vi "InstrPtr Demo.vi"() -> ()   [LabVIEW 2009]
uses:
  Dummy/Dummy.lvclass
  InstrPtr.lvclass
panel:
  out "*dummy":T1
  # "See block diagram."
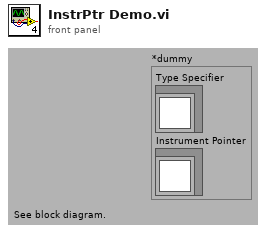
[diagram p1: front panel]
types:
  T1 = cluster{"Type Specifier":refnum<class "Dummy.lvclass">, "Instrument Pointer":refnum<class "InstrPtr.lvclass">}
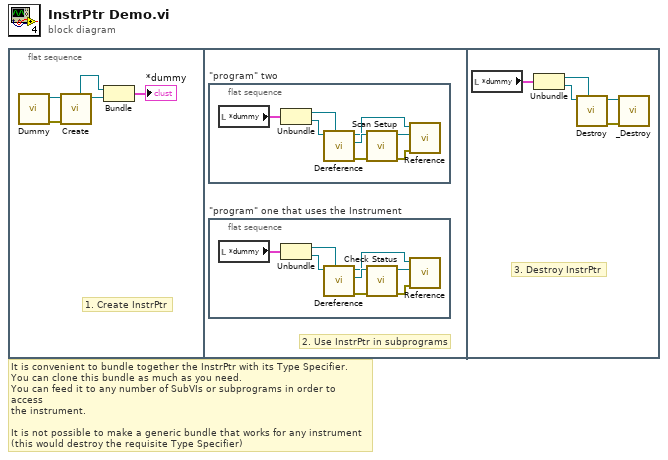
[diagram p0: block diagram]
diagram:
  # "It is convenient to bundle together the InstrPtr with its Type Specifier.\nYou can clone this bundle as much as you need.\nYou can feed it to any number of SubVIs or subprograms in order to access\nthe instrument.\n\nIt is not possible to make a generic bundle that works for any instrument\n(this would destroy the requisite Type Specifier)"
  n1 = flat-sequence {
    frame #0 {
      # "1. Create InstrPtr"
      n2 = call "Dummy.vi"() -> ("error out"=w5:errorcluster, "Dummy out"=w4:refnum<class "Dummy.lvclass">)  [unwired: 10 in]
      n3 = call "Create.vi"("error in (no error)"=w5, "Instrument in"=w4) -> ("Instrument Pointer"=w3:refnum<class "InstrPtr.lvclass">, "Type Specifier"=w2:refnum<class "Dummy.lvclass">)  [unwired: 1 in, 7 out]
      n4 = Bundle("Type Specifier"=w2, "Instrument Pointer"=w3) -> (→"*dummy":T1)  [unwired: 1 in]
    }
    frame #1 {
      # "2. Use InstrPtr in subprograms"
      n5 = flat-sequence "\"program\" two" {
        frame #0 {
          n6 = local read "*dummy"() -> (w9:T1)
          n7 = Unbundle(w9) -> ("Type Specifier"=w8:refnum<class "Dummy.lvclass">, "Instrument Pointer"=w7:refnum<class "InstrPtr.lvclass">)
          n8 = call "Dereference.vi"("Type Specifier"=w8, "InstrPtr"=w7) -> ("error out"=w13:errorcluster, "Instrument out"=w11:refnum<class "Dummy.lvclass">, "InstrPtr out"=w6:refnum<class "InstrPtr.lvclass">)  [unwired: 7 in]
          n9 = call-dynamic "Scan Setup.vi"("error in (no error)"=w13, "Instrument in"=w11) -> ("error out"=w12:errorcluster, "Instrument out"=w10:refnum<class "Dummy.lvclass">)  [unwired: 8 out]
          n10 = call "Reference.vi"("error in (no error)"=w12, "Instrument"=w10, "InstrPtr in"=w6) -> ()  [unwired: 8 in, 1 out]
        }
      }
      n11 = flat-sequence "\"program\" one that uses the Instrument" {
        frame #0 {
          n12 = local read "*dummy"() -> (w16:T1)
          n13 = Unbundle(w16) -> ("Type Specifier"=w15:refnum<class "Dummy.lvclass">, "Instrument Pointer"=w14:refnum<class "InstrPtr.lvclass">)
          n14 = call "Dereference.vi"("Type Specifier"=w15, "InstrPtr"=w14) -> ("error out"=w21:errorcluster, "Instrument out"=w19:refnum<class "Dummy.lvclass">, "InstrPtr out"=w17:refnum<class "InstrPtr.lvclass">)  [unwired: 7 in]
          n15 = call-dynamic "Check Status.vi"("error in (no error)"=w21, "Instrument in"=w19) -> ("error out"=w20:errorcluster, "Instrument out"=w18:refnum<class "Dummy.lvclass">)  [unwired: 8 out]
          n16 = call "Reference.vi"("error in (no error)"=w20, "Instrument"=w18, "InstrPtr in"=w17) -> ()  [unwired: 8 in, 1 out]
        }
      }
    }
    frame #2 {
      # "3. Destroy InstrPtr"
      n17 = local read "*dummy"() -> (w26:T1)
      n18 = Unbundle(w26) -> ("Type Specifier"=w25:refnum<class "Dummy.lvclass">, "Instrument Pointer"=w24:refnum<class "InstrPtr.lvclass">)
      n19 = call "Destroy.vi"("Type Specifier"=w25, "InstrPtr in"=w24) -> ("error out"=w22:errorcluster, "final Instrument"=w23:refnum<class "Dummy.lvclass">)  [unwired: 8 in]
      n20 = call-dynamic "_Destroy.vi"("error in (no error)"=w22, "Instrument in"=w23) -> ()  [unwired: 9 in, 1 out]
    }
  }
